vi "FTW-ActorRef-SpawnNewActor.vi"(0 "Actor Ref Prototype":refnum<class "FTW-ActorReference.lvclass">, 11 "error in":errorcluster) -> (4 "Actor Reference":refnum<class "FTW-ActorReference.lvclass">, 15 "error out":errorcluster)   [LabVIEW 2014, in "FTW-ActorReference.lvclass"]
uses:
  FTW-ActorReference.lvclass
  FTW-ActorReference.lvclass/FTW-ActorReference.ctl
  Context/FTW-Actor-Context.lvclass
  Context/Messaging/Address/FTW-Actor-Address.lvclass
panel:
  # "Inputs"
  # "Outputs"
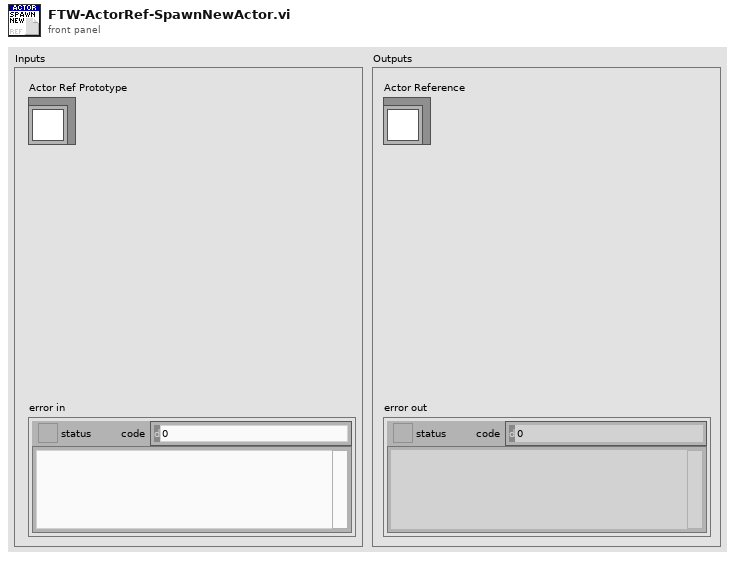
[diagram p1: front panel]
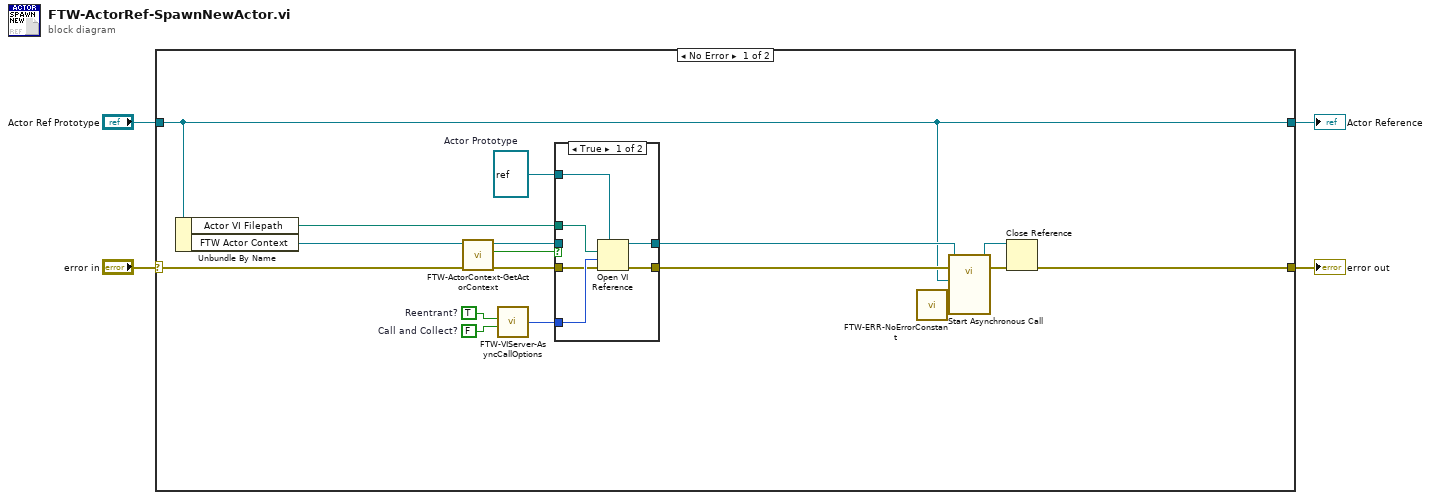
[diagram p0: block diagram]
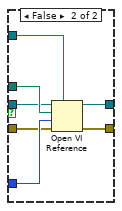
[diagram p2: hidden frame]
diagram:
  n1 = case shown="No Error" "error in" {
    selector: "error in" -> [w7 w36]
    tunnel: "Actor Ref Prototype" -> [w5 w35]
    tunnel: [w5 w35] -> w4
    tunnel: [w13 w36] -> w3
    frame No Error {
      w11 = refnum<vi> refnum  # Actor Prototype
      w18 = FALSE  # Call and Collect?
      w19 = TRUE  # Reentrant?
      n2 = Unbundle By Name(w5) -> ("Actor VI Filepath"=w12:path, "FTW Actor Context"=w10:refnum<class "FTW-Actor-Context.lvclass">)
      n3 = call "FTW-ActorContext-GetActorContext.vi"("error in"=w7, "Actor Context"=w10) -> ("error out"=w6:errorcluster, "Use Local Context"=w9:bool, "Actor Context"=w8:refnum<vi>)  [unwired: 7 in]
      n4 = call "FTW-VIServer-AsyncCallOptions.vi"("Call and Collect?"=w18, "Reentrant?"=w19) -> ("Open VI Ref Options"=w20:i32)  [unwired: 4 in]
      n5 = case shown="True" w9 {
        tunnel: [w27 w34] -> w21
        tunnel: w20 -> [w26 w33]
        tunnel: [w25 w32] -> w17
        tunnel: w8 -> [_ w28]
        tunnel: w6 -> [w24 w31]
        tunnel: w11 -> [w23 w30]
        tunnel: w12 -> [w22 w29]
        frame True {
          n6 = Open VI Reference(type specifier VI Refnum (for type only)=w23, vi path=w22, options=w26, error in (no error)=w24) -> (vi reference=w25:refnum<vi>, error out=w27:errorcluster)  [unwired: 2 in]
        }
        frame False {
          n7 = Open VI Reference(type specifier VI Refnum (for type only)=w30, application reference (local)=w28, vi path=w29, options=w33, error in (no error)=w31) -> (vi reference=w32:refnum<vi>, error out=w34:errorcluster)  [unwired: 1 in]
        }
      }
      n8 = call "FTW-ERR-NoErrorConstant.vi"() -> ("no error"=w14:errorcluster)
      n9 = call-by-ref "Start Asynchronous Call"(reference=w17, error in=w21, "Actor Ref Prototype"=w5, "error in"=w14) -> (reference out=w15:refnum<vi>, error out=w16:errorcluster)  [unwired: 13 in, 1 out]
      n10 = Close Reference(reference=w15, error in (no error)=w16) -> (error out=w13:errorcluster)
    }
    frame Error {
    }
  }
  "error out" <- w3
  "Actor Reference" <- w4
